vi "Game_Round.vi"(0 "Red Circle":refnum<vi>, 1 "ColorStr":refnum<vi>, 2 "Red Square":refnum<vi>, 3 "GreenSquare":refnum<vi>, 4 "ShapeStr":refnum<vi>, 5 "Green Circle":refnum<vi>) -> (6 "Elapsed Time":dbl, 7 "Correct Answer":bool, 8 "Valid Answer":bool)   [LabVIEW 2019]
uses:
  ButtonChoice.ctl
  Color.ctl
  Shape.ctl
  <vilib>/numeric/Random Number (Range) U64.vi
  <vilib>/numeric/Random Number (Range) I64.vi
  <vilib>/numeric/sub_Random U32.vi
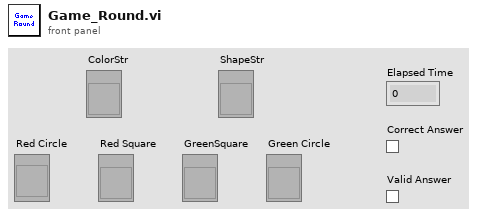
[diagram p1: front panel]
types:
  T1 = typedef "ButtonChoice.ctl" = cluster{"Color":T2, "Shape":T3}
  T2 = typedef "Color.ctl" = enum16{"Green", "Red"}
  T3 = typedef "Shape.ctl" = enum16{"Circle", "Square"}
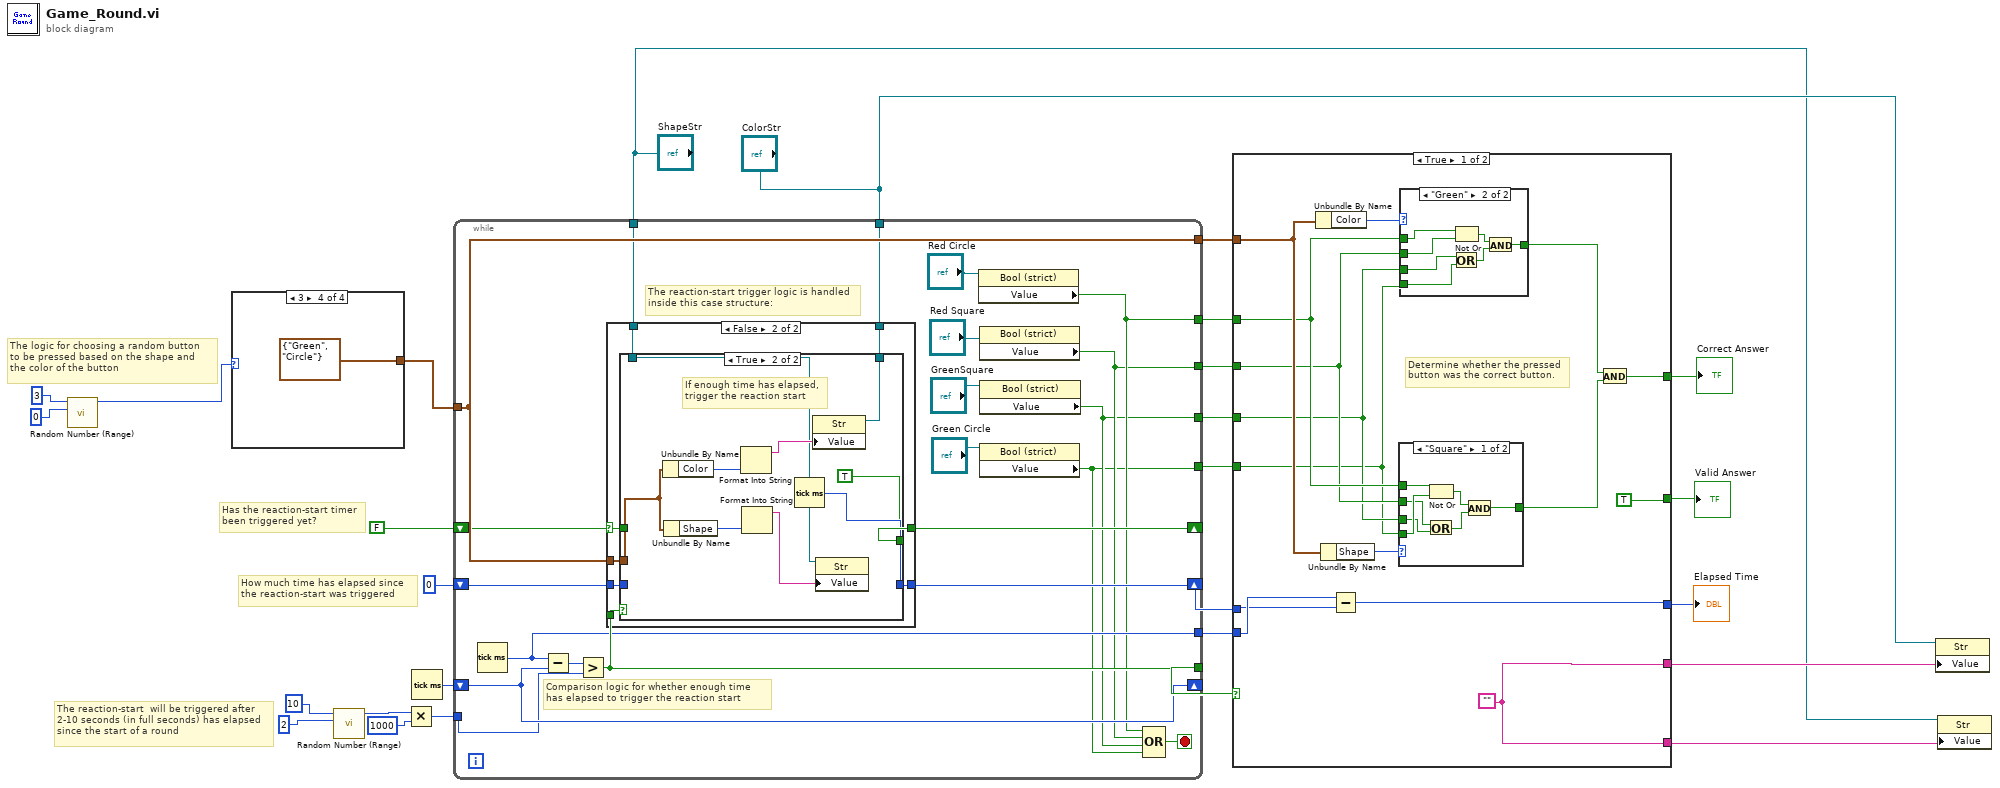
[diagram p0: block diagram]
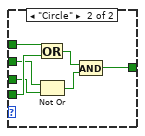
[diagram p2: hidden frame]
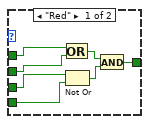
[diagram p3: hidden frame]
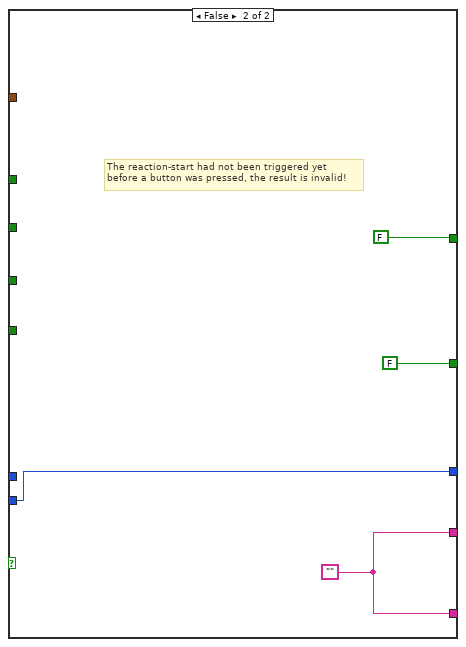
[diagram p4: hidden frame]
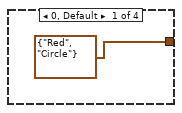
[diagram p5: hidden frame]
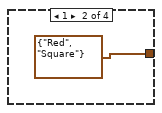
[diagram p6: hidden frame]
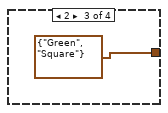
[diagram p7: hidden frame]
diagram:
  # "The logic for choosing a random button\nto be pressed based on the shape and\nthe color of the button"
  # "The reaction-start  will be triggered after \n2-10 seconds (in full seconds) has elapsed\nsince the start of a round"
  # "How much time has elapsed since\nthe reaction-start was triggered"
  # "Has the reaction-start timer\nbeen triggered yet?"
  n1 = call-poly <vilib>:"Random Number (Range).vi"("lower bound (-100)"=0, "upper bound (100)"=3) -> ("number"=w25:i64)  [unwired: 9 in]
  n2 = case shown="3" w25 {
    tunnel: [T1 {"Color"=enum."Red", "Shape"=enum."Circle"} ("Cluster") T1 {"Color"=enum."Red", "Shape"=enum."Square"} ("Cluster") T1 {"Color"=enum."Green", "Shape"=enum."Square"} ("Cluster") T1 {"Color"=enum."Green", "Shape"=enum."Circle"} ("Cluster")] -> w20
    frame 0, Default {
    }
    frame 1 {
    }
    frame 2 {
    }
    frame 3 {
    }
  }
  n3 = call-poly <vilib>:"Random Number (Range).vi"("lower bound (0)"=2, "upper bound (100)"=10) -> ("number"=w24:u64)  [unwired: 9 in]
  n4 = Multiply(x=w24, y=1000) -> (x*y=w19:u64)
  n5 = Tick Count (ms)() -> (millisecond timer value=w18:u32)
  n6 = while {
    tunnel: [w38] -> w16
    tunnel: [w36] -> w15
    tunnel: [w34] -> w14
    tunnel: [w32] -> w13
    tunnel: w20 -> [w48]
    tunnel: w19 -> [w50]
    shift-right: [w51] -> _
    shift-left: w18 -> [w51]
    tunnel: [w49] -> w17
    tunnel: [w48] -> w12
    tunnel: [w45] -> w11
    shift-right: [w46] -> w7
    shift-left: 0 -> [w44]
    shift-right: [w42] -> _
    shift-left: FALSE -> [w43]
    tunnel: "ColorStr" -> [w41]
    tunnel: "ShapeStr" -> [w40]
    stop <- w52 stop-if-true
    # "Comparison logic for whether enough time\nhas elapsed to trigger the reaction start"
    # "The reaction-start trigger logic is handled\ninside this case structure:"
    n7 = Tick Count (ms)() -> (millisecond timer value=w45:u32)
    n8 = Subtract(x=w45, y=w51) -> (x-y=w47:u32)
    n9 = Greater?(x=w47, y=w50) -> (0:w49:bool)
    n10 = case shown="False" w43 {
      selector: w43 -> [w54 w57]
      tunnel: w49 -> [_ w62]
      tunnel: w48 -> [_ w61]
      tunnel: [w53 w60] -> w46
      tunnel: w44 -> [w53 w59]
      tunnel: [w54 w58] -> w42
      tunnel: w41 -> [_ w56]
      tunnel: w40 -> [_ w55]
      frame True {
        # "The reaction-start Timer has already been triggered:\nDo nothing"
      }
      frame False {
        n11 = case shown="True" w62 {
          tunnel: w61 -> [_ w73]
          tunnel: [w64 w70] -> w60
          tunnel: w59 -> [w64 _]
          tunnel: [w63 TRUE] -> w58
          tunnel: w57 -> [w63 _]
          tunnel: w56 -> [_ w66]
          tunnel: w55 -> [_ w65]
          frame False {
          }
          frame True {
            # "If enough time has elapsed,\ntrigger the reaction start"
            n12 = Unbundle By Name(w73) -> ("Color"=w72:T2)
            n13 = Unbundle By Name(w73) -> ("Shape"=w71:T3)
            n14 = Format Into String(w72) -> (resulting string=w68:string)  [unwired: 3 in, 1 out]
            n15 = Format Into String(w71) -> (resulting string=w67:string)  [unwired: 3 in, 1 out]
            n16 = Tick Count (ms)() -> (millisecond timer value=w70:u32)
            n17 = property class="Str"(reference=w66, "Value"=w68) -> ()  [unwired: 1 in, 2 out]
            n18 = property class="Str"(reference=w65, "Value"=w67) -> ()  [unwired: 1 in, 2 out]
          }
        }
      }
    }
    n19 = property class="Bool (strict)"(reference="Red Circle") -> ("Value"=w38:bool)  [unwired: 1 in, 2 out]
    n20 = property class="Bool (strict)"(reference="Red Square") -> ("Value"=w36:bool)  [unwired: 1 in, 2 out]
    n21 = property class="Bool (strict)"(reference="Green Circle") -> ("Value"=w32:bool)  [unwired: 1 in, 2 out]
    n22 = property class="Bool (strict)"(reference="GreenSquare") -> ("Value"=w34:bool)  [unwired: 1 in, 2 out]
    n23 = Compound Arithmetic op=OR(w38, w36, w34, w32) -> (w52:bool)
  }
  n24 = case shown="True" w17 {
    tunnel: [w74 w117] -> w4
    tunnel: [w74 w117] -> w1
    tunnel: w16 -> [w85 _]
    tunnel: w15 -> [w84 _]
    tunnel: w14 -> [w83 _]
    tunnel: w13 -> [w82 _]
    tunnel: w12 -> [w88 _]
    tunnel: w11 -> [w77 w119]
    tunnel: [w75 w119] -> w10
    tunnel: [w79 FALSE] -> w9
    tunnel: [TRUE FALSE] -> w8
    tunnel: w7 -> [w76 _]
    frame True {
      w74 = ""
      # "Determine whether the pressed\nbutton was the correct button."
      n25 = Unbundle By Name(w88) -> ("Color"=w87:T2)
      n26 = Unbundle By Name(w88) -> ("Shape"=w86:T3)
      n27 = Subtract(x=w77, y=w76) -> (x-y=w75:u32)
      n28 = case shown="\"Square\"" w86 {
        tunnel: w85 -> [w92 w99]
        tunnel: w84 -> [w90 w97]
        tunnel: w83 -> [w89 w96]
        tunnel: w82 -> [w91 w98]
        tunnel: [w95 w102] -> w80
        frame "Square" {
          n29 = Not Or(1:w91, 2:w92) -> (0:w93:bool)
          n30 = Or(x=w90, y=w89) -> (x .or. y?=w94:bool)
          n31 = And(x=w93, y=w94) -> (x .and. y?=w95:bool)
        }
        frame "Circle" {
          n32 = Or(x=w99, y=w98) -> (x .or. y?=w100:bool)
          n33 = Not Or(1:w96, 2:w97) -> (0:w101:bool)
          n34 = And(x=w100, y=w101) -> (x .and. y?=w102:bool)
        }
      }
      n35 = case shown="\"Green\"" w87 {
        tunnel: w85 -> [w104 w113]
        tunnel: w84 -> [w103 w112]
        tunnel: w83 -> [w106 w111]
        tunnel: w82 -> [w105 w110]
        tunnel: [w107 w114] -> w81
        frame "Red" {
          n36 = Or(x=w104, y=w103) -> (x .or. y?=w109:bool)
          n37 = Not Or(1:w105, 2:w106) -> (0:w108:bool)
          n38 = And(x=w109, y=w108) -> (x .and. y?=w107:bool)
        }
        frame "Green" {
          n39 = Not Or(1:w112, 2:w113) -> (0:w116:bool)
          n40 = Or(x=w111, y=w110) -> (x .or. y?=w115:bool)
          n41 = And(x=w116, y=w115) -> (x .and. y?=w114:bool)
        }
      }
      n42 = And(x=w81, y=w80) -> (x .and. y?=w79:bool)
    }
    frame False {
      w117 = ""
      # "The reaction-start had not been triggered yet\nbefore a button was pressed, the result is invalid!"
    }
  }
  "Elapsed Time" <- w10
  "Correct Answer" <- w9
  "Valid Answer" <- w8
  n43 = property class="Str"(reference="ColorStr", "Value"=w4) -> ()  [unwired: 1 in, 2 out]
  n44 = property class="Str"(reference="ShapeStr", "Value"=w1) -> ()  [unwired: 1 in, 2 out]
